vi "Connect.vi"(8 "error in (no error)":errorcluster, 10 "URL":string, 11 "Client In":refnum<class "Client.lvclass">) -> (0 "error out":errorcluster, 2 "ret":i32, 3 "Client out":refnum<class "Client.lvclass">)   [LabVIEW 2017, in "opcua.lvlib" / "Client.lvclass"]
uses:
  Client.lvclass
  Client.lvclass/Client.ctl
  opcua32.dll
  opcua.lvlib
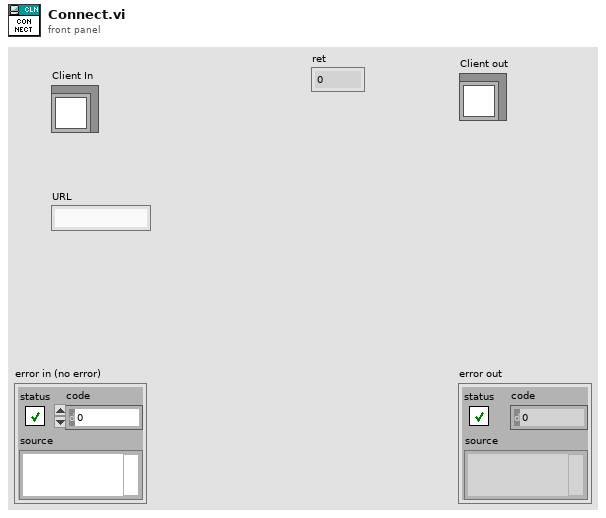
[diagram p1: front panel]
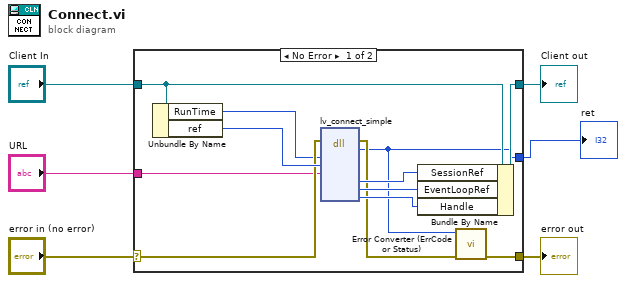
[diagram p0: block diagram]
diagram:
  n1 = case shown="No Error" "error in (no error)" {
    selector: "error in (no error)" -> [w13 w19]
    tunnel: [w8 w19] -> w5
    tunnel: [w18 w20] -> w4
    tunnel: "Client In" -> [w17 w20]
    tunnel: "URL" -> [w12 _]
    tunnel: [w7 _] -> w1
    frame No Error {
      n2 = Unbundle By Name(w17) -> ("RunTime"=w11:u64, "ref"=w16:u64)
      n3 = dll-call lib="C:/Users/Andrey/Desktop/opcua-labview/opcua-lvlib/opcua*.dll" fn="lv_connect_simple"(error in=w13, "RunTime"=w11, "client_ref"=w16, "URL"=w12) -> (error out=w9:errorcluster, "return type"=w7:i32, "SessionRefOut"=w15:u64, "EventLoopRefOut"=w14:u64, "Handle"=w10:u64)  [unwired: 8 in, 1 out]
      n4 = Bundle By Name(cluster=w17, "SessionRef"=w15, "EventLoopRef"=w14, "Handle"=w10) -> (w18:refnum<class "Client.lvclass">)
      n5 = call "Error Converter (ErrCode or Status).vi"("error in (no error)"=w9, "error code"=w7) -> ("error out"=w8:errorcluster)  [unwired: 9 in]
    }
    frame Error {
    }
  }
  "error out" <- w5
  "Client out" <- w4
  "ret" <- w1
